vi "Stop Everything.vi"(8 "error in":errorcluster, 11 "TCP slave instance":refnum<class "Modbus Slave.lvclass">) -> (0 "error out":errorcluster, 3 "TCP slave instance":refnum<class "Modbus Slave.lvclass">)   [LabVIEW 2021]
uses:
  <vilib>/Modbus/slave/Modbus Slave.lvclass
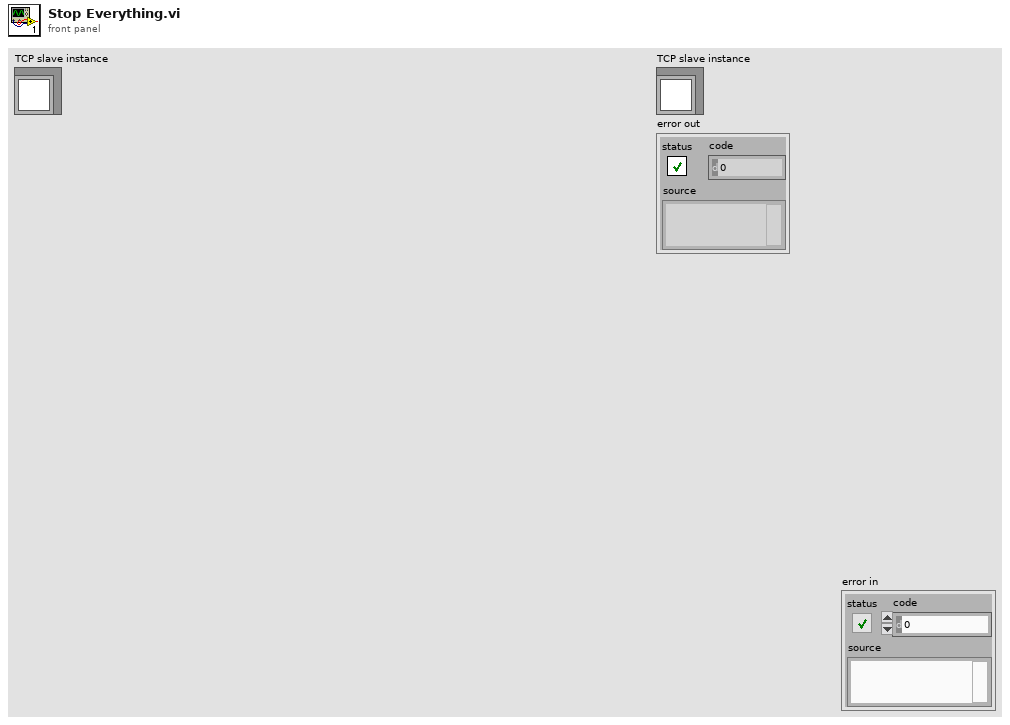
[diagram p1: front panel]
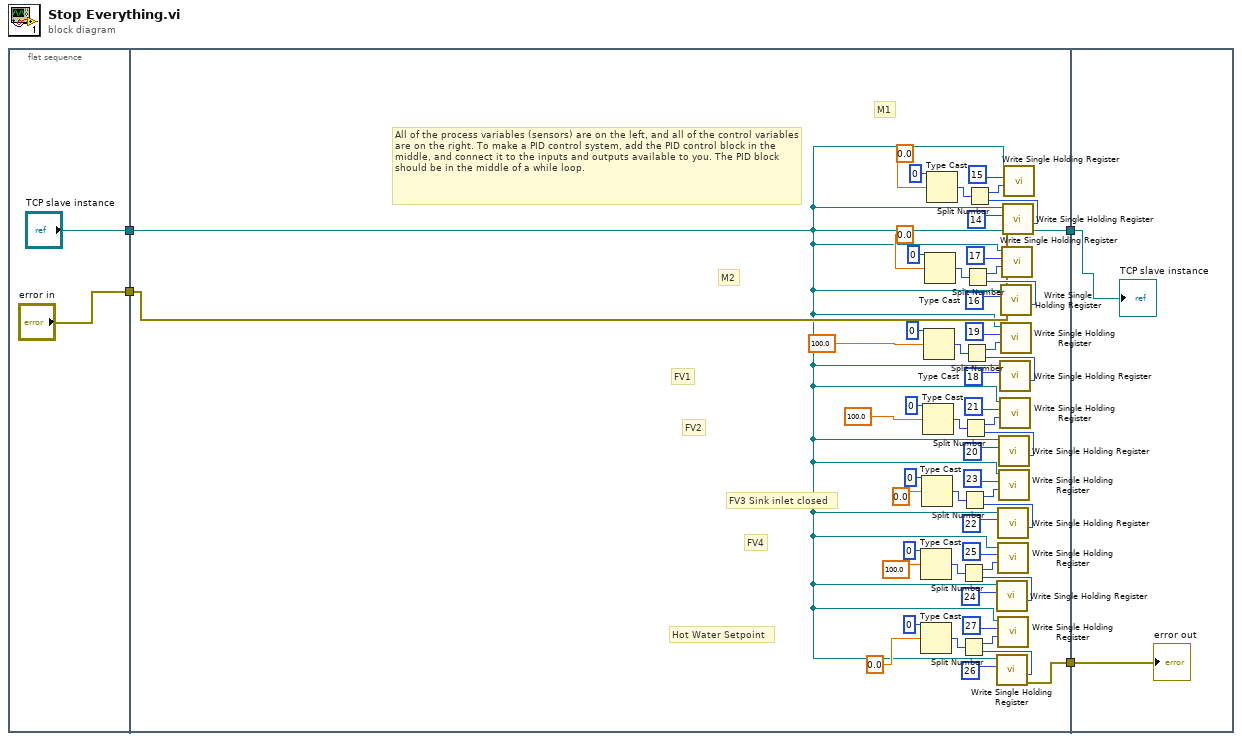
[diagram p0: block diagram]
diagram:
  n1 = flat-sequence {
    tunnel: ["error in"] -> w4
    tunnel: ["TCP slave instance"] -> w3
    tunnel: w4 -> [w9]
    tunnel: [w8] -> w2
    tunnel: w3 -> [w8]
    tunnel: [w7] -> w1
    tunnel: w2 -> [w60]
    tunnel: w1 -> [w59]
    frame #0 {
    }
    frame #1 {
      # "Hot Water Setpoint"
      # "FV4"
      # "FV3 Sink inlet closed"
      # "FV2"
      # "FV1"
      # "M2"
      # "M1"
      # "All of the process variables (sensors) are on the left, and all of the control variables are on the right. To make a PID control system, add the PID control block in the middle, and connect it to the inputs and outputs available to you. The PID block should be in the middle of a while loop."
      n2 = Type Cast(type=u32 0, x=sgl 100.0 ("FV4")) -> (*(type *) &x=w19:u32)
      n3 = Type Cast(type=u32 0, x=sgl 0.0 ("Hot Water Setpoint")) -> (*(type *) &x=w12:u32)
      n4 = Type Cast(type=u32 0, x=sgl 0.0 ("FV3")) -> (*(type *) &x=w26:u32)
      n5 = Type Cast(type=u32 0, x=sgl 100.0 ("FV2")) -> (*(type *) &x=w33:u32)
      n6 = Type Cast(type=u32 0, x=sgl 100.0 ("FV1")) -> (*(type *) &x=w40:u32)
      n7 = Type Cast(type=u32 0, x=sgl 0.0 ("M2")) -> (*(type *) &x=w47:u32)
      n8 = Type Cast(type=u32 0, x=sgl 0.0 ("M1")) -> (*(type *) &x=w54:u32)
      n9 = Split Number(x=w19) -> (hi(x)=w21:u16, lo(x)=w20:u16)
      n10 = Split Number(x=w12) -> (hi(x)=w14:u16, lo(x)=w13:u16)
      n11 = Split Number(x=w26) -> (hi(x)=w28:u16, lo(x)=w27:u16)
      n12 = Split Number(x=w33) -> (hi(x)=w35:u16, lo(x)=w34:u16)
      n13 = Split Number(x=w40) -> (hi(x)=w42:u16, lo(x)=w41:u16)
      n14 = Split Number(x=w47) -> (hi(x)=w49:u16, lo(x)=w48:u16)
      n15 = Split Number(x=w54) -> (hi(x)=w56:u16, lo(x)=w55:u16)
      n16 = call-dynamic "Write Single Holding Register.vi"("holding register value"=w20, "address"=u16 24, "Modbus slave in"=w8) -> ()  [unwired: 7 in, 2 out]
      n17 = call-dynamic "Write Single Holding Register.vi"("holding register value"=w13, "address"=u16 26, "Modbus slave in"=w8) -> ("error out"=w7:errorcluster)  [unwired: 7 in, 1 out]
      n18 = call-dynamic "Write Single Holding Register.vi"("holding register value"=w27, "address"=u16 22, "Modbus slave in"=w8) -> ()  [unwired: 7 in, 2 out]
      n19 = call-dynamic "Write Single Holding Register.vi"("holding register value"=w21, "address"=u16 25, "Modbus slave in"=w8) -> ()  [unwired: 7 in, 2 out]
      n20 = call-dynamic "Write Single Holding Register.vi"("holding register value"=w14, "address"=u16 27, "Modbus slave in"=w8) -> ()  [unwired: 7 in, 2 out]
      n21 = call-dynamic "Write Single Holding Register.vi"("holding register value"=w34, "address"=u16 20, "Modbus slave in"=w8) -> ()  [unwired: 7 in, 2 out]
      n22 = call-dynamic "Write Single Holding Register.vi"("holding register value"=w28, "address"=u16 23, "Modbus slave in"=w8) -> ()  [unwired: 7 in, 2 out]
      n23 = call-dynamic "Write Single Holding Register.vi"("holding register value"=w41, "address"=u16 18, "Modbus slave in"=w8) -> ()  [unwired: 7 in, 2 out]
      n24 = call-dynamic "Write Single Holding Register.vi"("holding register value"=w35, "address"=u16 21, "Modbus slave in"=w8) -> ()  [unwired: 7 in, 2 out]
      n25 = call-dynamic "Write Single Holding Register.vi"("holding register value"=w48, "address"=u16 16, "Modbus slave in"=w8) -> ()  [unwired: 7 in, 2 out]
      n26 = call-dynamic "Write Single Holding Register.vi"("holding register value"=w42, "address"=u16 19, "Modbus slave in"=w8) -> ()  [unwired: 7 in, 2 out]
      n27 = call-dynamic "Write Single Holding Register.vi"("holding register value"=w49, "address"=u16 17, "Modbus slave in"=w8) -> ()  [unwired: 7 in, 2 out]
      n28 = call-dynamic "Write Single Holding Register.vi"("error in (no error)"=w9, "holding register value"=w55, "address"=u16 14, "Modbus slave in"=w8) -> ()  [unwired: 6 in, 2 out]
      n29 = call-dynamic "Write Single Holding Register.vi"("holding register value"=w56, "address"=u16 15, "Modbus slave in"=w8) -> ()  [unwired: 7 in, 2 out]
    }
    frame #2 {
      "TCP slave instance" <- w60
      "error out" <- w59
    }
  }
